vi "ConfirmFile.vi"(3 "Error In":errorcluster, 4 "Filename IN":string, 5 "Pathname IN":string) -> (0 "Error Out":errorcluster, 1 "Run Number":i32, 2 "Filename:":string)   [LabVIEW 2013]
uses:
  globals/QC_RunInformation.vi
panel:
  out "Pathname":string
  out "Folder already existed":bool
  in  "stop":bool
  # "Saving Data File"
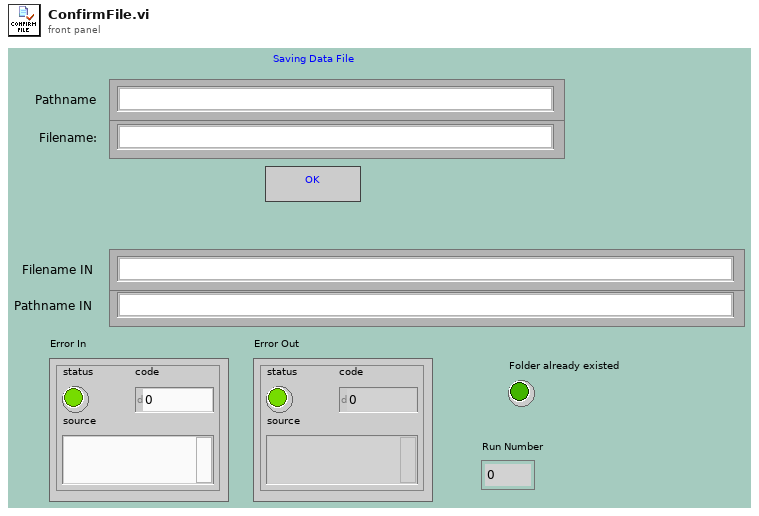
[diagram p1: front panel]
types:
  T1 = cluster{"Sensor Serial No.:":string, "Wafer:":string, "Batch:":string, "Manufacturer:":string, "Device Category:":string, "Database Serial No.:":string, "Date Initiated:":string, "Time Initiated:":string, "Test":string, "Probeplan used:":string, "End of Run comment:":string, "User:":string, "Vbias SMU":string, "LCR":string, "Test SMU":string, "Test DMM":string}
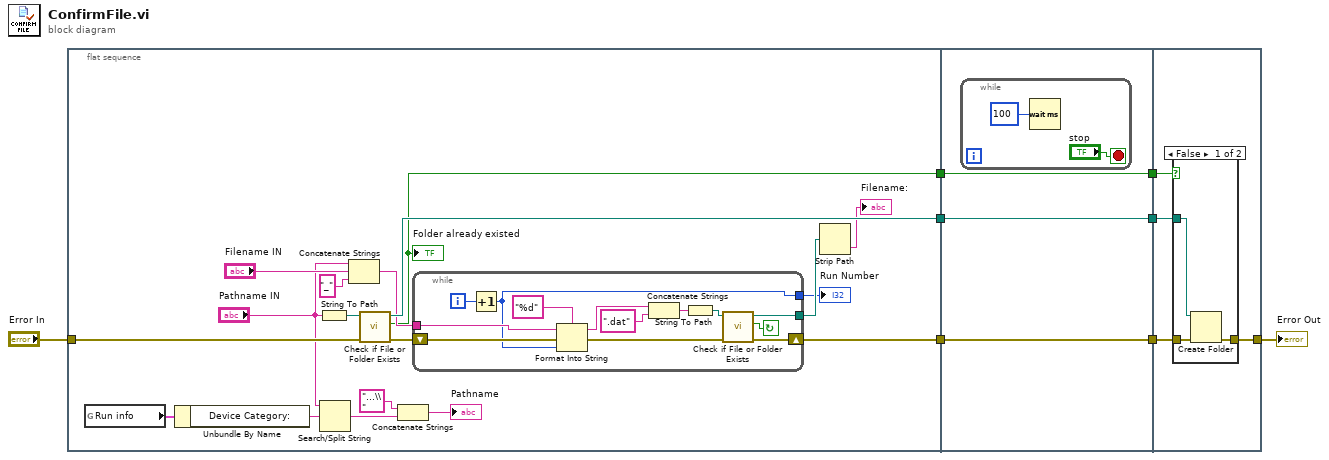
[diagram p0: block diagram]
diagram:
  n1 = flat-sequence {
    tunnel: "Error In" -> [w26]
    tunnel: [w21] -> w5
    tunnel: [w24] -> w4
    tunnel: [w19] -> w2
    tunnel: [w42] -> w6
    tunnel: w5 -> [w42]
    tunnel: w4 -> [w41]
    tunnel: [w41] -> w3
    tunnel: w2 -> [w40]
    tunnel: [w40] -> w1
    tunnel: [w48] -> w7
    tunnel: w6 -> [w47]
    tunnel: w3 -> [w46]
    tunnel: w1 -> [w45]
    frame #0 {
      n2 = global read "QC_RunInformation.vi" "Run info"() -> (w14:T1)
      n3 = Unbundle By Name(w14) -> ("Device Category:"=w13:string)
      n4 = String To Path(string="Pathname IN") -> (path=w25:path)
      n5 = Search/Split String(string="Pathname IN", search string/char (-)=w13) -> (match + rest of string=w11:string)  [unwired: 1 in, 2 out]
      n6 = Concatenate Strings("Pathname IN", "Filename IN", "_") -> (w20:string)
      n7 = call <vilib>:"Check if File or Folder Exists.vi"("error in (no error)"=w26, "path"=w25) -> ("error out"=w22:errorcluster, "file or folder exists?"=w19:bool, "dup path"=w24:path)  [unwired: 7 in]
      "Folder already existed" <- w19
      n8 = Concatenate Strings("...\\", w11) -> (→"Pathname":string)
      n9 = while {
        shift-right: [w38] -> w21
        shift-left: w22 -> [w33]
        tunnel: w20 -> [w36]
        tunnel: [w31] -> w17
        tunnel: [w27] -> w9
        i -> [w37]
        stop <- w39 continue-if-true
        n10 = Increment(x=w37) -> (x+1=w27:i32)
        n11 = Format Into String(format string="%d", initial string=w36, error in=w33, w27) -> (resulting string=w30:string, error out=w32:errorcluster)
        n12 = Concatenate Strings(w30, ".dat") -> (w28:string)
        n13 = String To Path(string=w28) -> (path=w34:path)
        n14 = call <vilib>:"Check if File or Folder Exists.vi"("error in (no error)"=w32, "path"=w34) -> ("error out"=w38:errorcluster, "file or folder exists?"=w39:bool, "dup path"=w31:path)  [unwired: 7 in]
      }
      "Run Number" <- w9
      n15 = Strip Path(path=w17) -> (name=→"Filename:":string)  [unwired: 1 out]
    }
    frame #1 {
      n16 = while {
        stop <- "stop" stop-if-true
        n17 = Wait (ms)(milliseconds to wait=u32 100) -> ()  [unwired: 1 out]
      }
    }
    frame #2 {
      n18 = case shown="False" w45 {
        tunnel: w47 -> [w51 w52]
        tunnel: w46 -> [w50 _]
        tunnel: [w49 w52] -> w48
        frame False {
          n19 = Create Folder(path (use dialog)=w50, error in=w51) -> (error out=w49:errorcluster)  [unwired: 1 in, 2 out]
        }
        frame True {
        }
      }
    }
  }
  "Error Out" <- w7
